vi "Read Temperature (C).vi"(8 "error in (no error)":errorcluster, 11 "LPS Barometric Pressure Sensor in":refnum<class "LPS Barometric Pressure Sensor.lvclass">) -> (0 "error out":errorcluster, 2 "Temperature (degC)":dbl, 3 "LPS Barometric Pressure Sensor out":refnum<class "LPS Barometric Pressure Sensor.lvclass">)   [LabVIEW 2020, in "LPS Barometric Pressure Sensor.lvclass"]
doc: "Reads the temperature in degrees Celsius (C)."
uses:
  LPS Barometric Pressure Sensor.lvclass
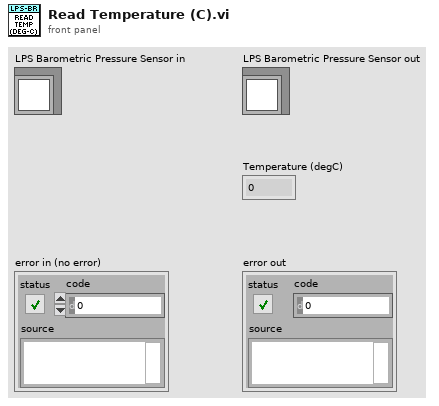
[diagram p1: front panel]
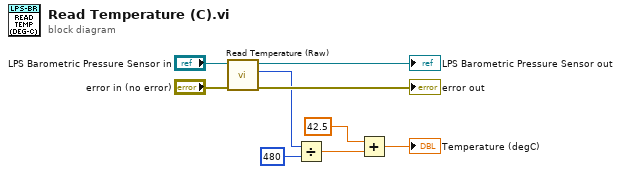
[diagram p0: block diagram]
diagram:
  n1 = call-dynamic "Read Temperature (Raw).vi"("error in (no error)"="error in (no error)", "LPS Barometer in"="LPS Barometric Pressure Sensor in") -> ("error out"=→"error out":errorcluster, "Raw Temperature"=w5:i16, "LPS Barometer out"=→"LPS Barometric Pressure Sensor out":refnum<class "LPS Barometric Pressure Sensor.lvclass">)  [unwired: 7 in]
  n2 = Divide(x=w5, y=i16 480) -> (x/y=w3:dbl)
  n3 = Add(x=42.5, y=w3) -> (x+y=→"Temperature (degC)":dbl)
